vi "Switch_MotorP5_GetAttributes.vi"(8 "error in (no error)":errorcluster, 10 "OnlyGetDvrReference(False)":bool, 11 "reference in":refnum<class "Switch_MotorP5.lvclass">) -> (0 "error out":errorcluster, 1 "DataRef":refnum<data-value>, 2 "Data":T1={"Config"={"COM"="", "SwitchMap"=[], "Sim"=FALSE}, "VISA"="", "RPM"=0, "States"=[], "UpdateEvent"=refnum, "Motor"=enum."M7"}, 3 "reference out":refnum<class "Switch_MotorP5.lvclass">)   [LabVIEW 2022 SP3, in "Switch_MotorP5.lvlib" / "Switch_MotorP5.lvclass"]
uses:
  Switch_MotorP5.lvclass
  protected/ObjectAttributes.ctl
  protected/Config.ctl
  Switch_MotorP5.lvclass/Switch_MotorP5.ctl
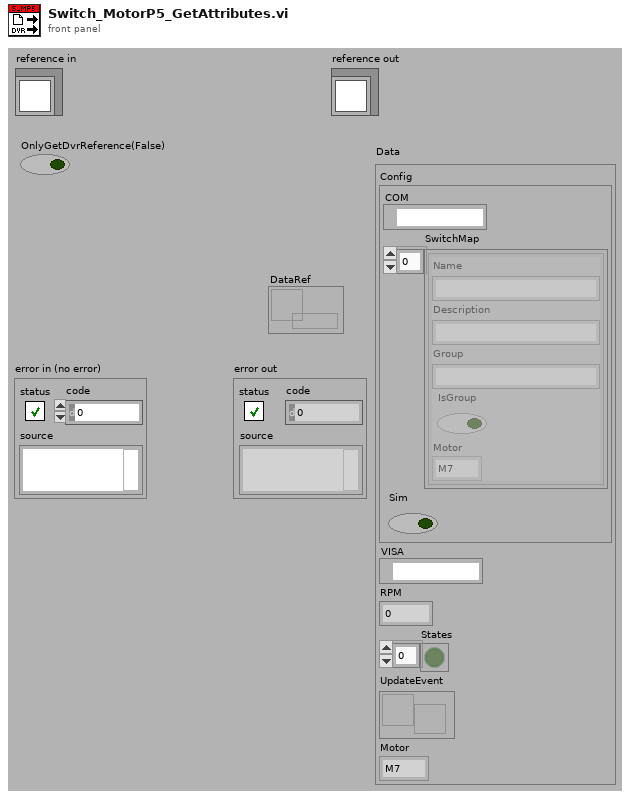
[diagram p1: front panel]
types:
  T1 = typedef "Switch_MotorP5.lvlib/Switch_MotorP5.lvclass/ObjectAttributes.ctl" = cluster{"Config":T2, "VISA":refnum<visa-resource-name>, "RPM":i32, "States":bool[], "UpdateEvent":refnum<user-event>, "Motor":enum32{"M1", "M2", "M3", "M4", "M5", "M6", "M7", "M8"}}
  T2 = typedef "Switch_MotorP5.lvlib/Switch_MotorP5.lvclass/Config.ctl" = cluster{"COM":refnum<visa-resource-name>, "SwitchMap":cluster{"Name":string, "Description":string, "Group":string, "IsGroup":bool, "Motor":enum32{"M1", "M2", "M3", "M4", "M5", "M6", "M7", "M8", "NA"}}[], "Sim":bool}
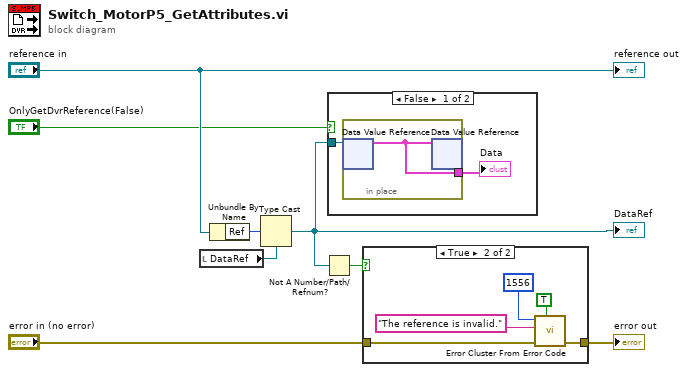
[diagram p0: block diagram]
diagram:
  n1 = local read "DataRef"() -> (w2:refnum<data-value>)
  n2 = Unbundle By Name("reference in") -> ("Ref"=w3:u32)
  n3 = Type Cast(type=w2, x=w3) -> (*(type *) &x=w5:refnum<data-value>)
  "DataRef" <- w5
  n4 = Not A Number/Path/Refnum?(number/path/refnum=w5) -> (NaN/Path/Refnum?=w1:bool)
  n5 = case shown="False" "OnlyGetDvrReference(False)" {
    tunnel: w5 -> [w10 _]
    frame False {
      n6 = in-place {
        in-place-border: [w11] -> w9
        n7 = in-place-dvr #1(w10) -> (w11:T1)  [unwired: 1 out]
        n8 = in-place-dvr #1(w11) -> ()  [unwired: 2 out]
      }
      "Data" <- w9
    }
    frame True {
    }
  }
  n9 = case shown="True" w1 {
    tunnel: "error in (no error)" -> [w12 w14]
    tunnel: [w12 w13] -> w7
    frame False {
    }
    frame True {
      n10 = call <vilib>:"Error Cluster From Error Code.vi"("show call chain? (False)"=TRUE, "error in (no error)"=w14, "error message (\"\")"="The reference is invalid." ("source"), "error code (0)"=1556 ("code")) -> ("error out"=w13:errorcluster)  [unwired: 5 in]
    }
  }
  "error out" <- w7
  "reference out" <- "reference in"
